vi "pcbPositioning.vi"() -> ()   [LabVIEW 2011]
panel:
  in  "PCB 1":dbl
  in  "aspirazione":bool caption="Posizionare i perni di centraggio dei PCB"
  in  "centraggioPCB":bool caption="Posizionare i perni di centraggio dei PCB"
  in  "PCB":bool caption="Posizionare i PCB sulle piastre tavolo"
  in  "ptfe":bool caption="Posizionare i perni di centraggio cornici in teflon sulle piastre tavolo"
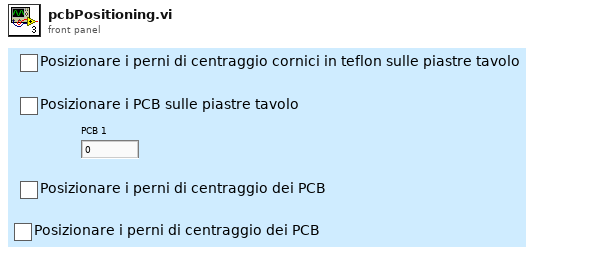
[diagram p1: front panel]
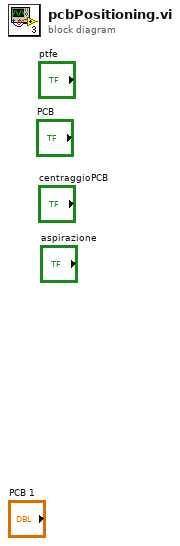
[diagram p0: block diagram]
diagram:
